vi "Parse Packet Data (Error).vi"(8 "error in (no error)":errorcluster, 10 "Recieved Bytes":u8[](array[numeric])) -> (0 "error out":errorcluster)   [LabVIEW 2014, in "hse-db.lvlib" / "MySQL (TCP).lvlib"]
uses:
  MySQL (TCP).lvlib
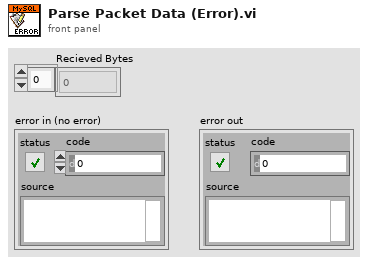
[diagram p1: front panel]
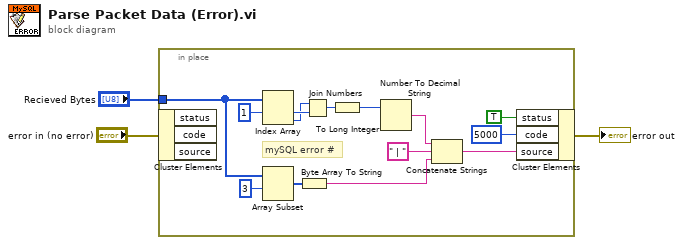
[diagram p0: block diagram]
diagram:
  n1 = in-place {
    in-place-border: "Recieved Bytes" -> [w13]
    # "mySQL error #"
    n2 = in-place-cluster #1("error in (no error)") -> ()  [unwired: 3 out]
    n3 = Index Array(array=w13, index #1=1 ("index")) -> (element #1=w8:u8, element #2=w7:u8)  [unwired: 1 in]
    n4 = Array Subset(array=w13, index=3) -> (w12:u8[])  [unwired: 1 in]
    n5 = Byte Array To String(unsigned byte array=w12) -> (string=w14:string)
    n6 = Join Numbers(hi=w7, lo=w8) -> ((hi.lo)=w9:u16)
    n7 = To Long Integer(number=w9) -> (32bit integer=w16:i32)
    n8 = Number To Decimal String(number=w16) -> (decimal integer string=w17:string)  [unwired: 1 in]
    n9 = Concatenate Strings(w17, " | " ("string"), w14) -> (w6:string)
    n10 = in-place-cluster #1("status"=TRUE, "code"=5000, "source"=w6) -> (→"error out":errorcluster)
  }
